vi "log_controls.vi"(0 "Controls[]":refnum<vi>[](array[refnum]), 2 "filename":path) -> (8 "error out":errorcluster)   [LabVIEW 2015]
doc: "Copyright (c) 2018 Frans Korhonen, Institute for Atmospheric and Earth System Research / Physics, Faculty of Science, University of Helsinki, Finland\n\nThis file is part of MeasGUI.\n\nThis Source Code Form is subject to the terms of the Mozilla Public\nLicense, v. 2.0. If a copy of the MPL was not distributed with this\n file, You can obtain one at http://mozilla.org/MPL/2.0/."
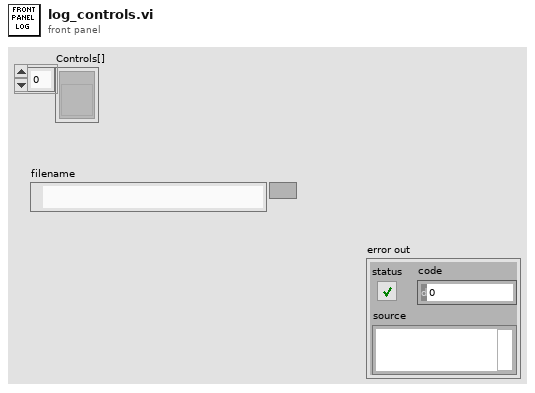
[diagram p1: front panel]
types:
  T1 = enum16{"open", "replace", "create", "open or create", "replace or create", "replace or create with confirmation"}
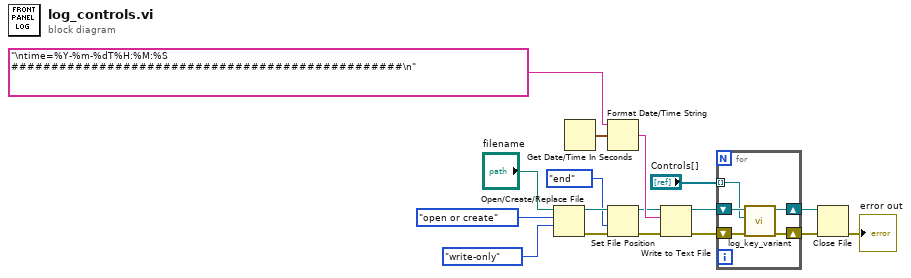
[diagram p0: block diagram]
diagram:
  n1 = Open/Create/Replace File(file path (use dialog)="filename", operation (0:open)=T1."open or create", access (0:read/write)=enum16{"read/write", "read-only", "write-only"}."write-only") -> (refnum out=w7:refnum<file>, error out=w8:errorcluster)  [unwired: 3 in, 1 out]
  n2 = Get Date/Time In Seconds() -> (seconds since 1Jan1904=w12:timestamp)
  n3 = Format Date/Time String(time format string (%c)="\ntime=%Y-%m-%dT%H:%M:%S #################################################\n", seconds (now)=w12) -> (date/time string=w10:string)  [unwired: 1 in]
  n4 = Set File Position(refnum=w7, from (0:start)=enum16{"start", "end", "current"}."end", error in=w8) -> (refnum out=w6:refnum<file>, error out=w5:errorcluster)  [unwired: 1 in]
  n5 = Write to Text File(file (use dialog)=w6, text=w10, error in=w5) -> (refnum out=w3:refnum<file>, error out=w9:errorcluster)  [unwired: 1 in, 1 out]
  n6 = for {
    shift-right: [w19] -> w2
    shift-left: w3 -> [w20]
    shift-right: [w22] -> w16
    shift-left: w9 -> [w21]
    tunnel: "Controls[]" -> [w18] mode=indexing
    n7 = call "log_key_variant.vi"("error in (no error)"=w21, "Ctl Refnum"=w18, "Byte Stream File in"=w20) -> ("error out"=w22:errorcluster, "Byte Stream File out"=w19:refnum<file>)  [unwired: 7 in]
  }
  n8 = Close File(refnum=w2, error in=w16) -> (error out=→"error out":errorcluster)  [unwired: 1 out]
